vi "tt20panel_DO_apply_settings.vi"(8 "error in (no error)":errorcluster, 10 "tt20_settings":T1, 11 "tt20panel in":refnum<class "tt20panel.lvclass">) -> (0 "error out":errorcluster, 3 "tt20panel out":refnum<class "tt20panel.lvclass">)   [LabVIEW 2015, in "tt20panel.lvclass"]
uses:
  tt20panel.lvclass
  tt20_class/tt20_hardware_info_tdef.ctl
  tt20_acq_mode_tdef.ctl
  tt20_class/tt20.lvclass
  UI/panel_class/panel.lvclass
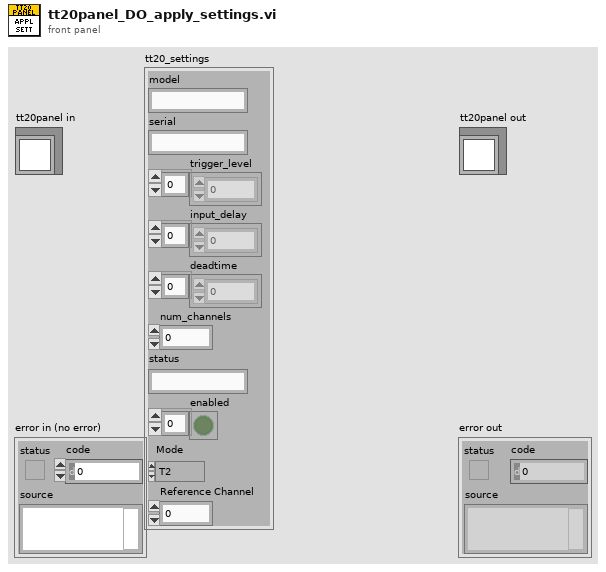
[diagram p1: front panel]
types:
  T1 = typedef "tt20_hardware_info_tdef.ctl" = cluster{"model":string, "serial":string, "trigger_level":dbl[], "input_delay":i64[], "deadtime":i64[], "num_channels":u32, "status":string, "enabled":bool[], "Mode":T2, "Reference Channel":u8}
  T2 = typedef "tt20_acq_mode_tdef.ctl" = enum16{"T2", "T3"}
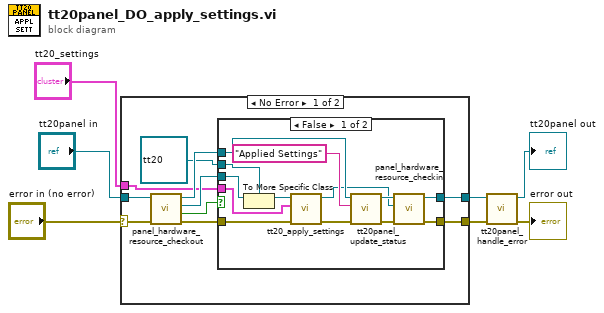
[diagram p0: block diagram]
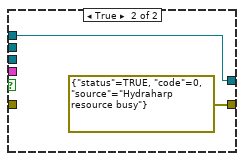
[diagram p2: hidden frame]
diagram:
  n1 = case shown="No Error" "error in (no error)" {
    selector: "error in (no error)" -> [w16 w34]
    tunnel: [w13 w34] -> w5
    tunnel: [w10 w33] -> w2
    tunnel: "tt20panel in" -> [w17 w33]
    tunnel: "tt20_settings" -> [w8 _]
    frame No Error {
      n2 = call "panel_hardware_resource_checkout.vi"("error in (no error)"=w16, "panel in"=w17) -> ("error out"=w14:errorcluster, "timed out?"=w15:bool, "hardware.lvclass"=w11:refnum<class "hardware.lvclass">, "panel out"=w12:refnum<class "tt20panel.lvclass">)  [unwired: 6 in]
      n3 = case shown="False" w15 {
        tunnel: w14 -> [w22 _]
        tunnel: [w28 errorcluster {"status"=TRUE, "code"=0, "source"="Hydraharp resource busy"} ("error out")] -> w13
        tunnel: w12 -> [w26 w31]
        tunnel: w11 -> [w29 _]
        tunnel: refnum<class "tt20.lvclass"> refnum ("tt20.lvclass") -> [w30 _]
        tunnel: [w27 w31] -> w10
        tunnel: w8 -> [w18 _]
        frame False {
          n4 = To More Specific Class(target class=w30, reference=w29) -> (specific class reference=w19:refnum<class "tt20.lvclass">)  [unwired: 1 in, 1 out]
          n5 = call "tt20_apply_settings.vi"("error in (no error)"=w22, "tt20_info"=w18, "tt20 in"=w19) -> ("error out"=w21:errorcluster, "tt20 out"=w20:refnum<class "tt20.lvclass">)  [unwired: 7 in]
          n6 = call "tt20panel_update_status.vi"("error in (no error)"=w21, "status"="Applied Settings", "tt20panel in"=w26) -> ("error out"=w24:errorcluster, "tt20panel out"=w25:refnum<class "tt20panel.lvclass">)  [unwired: 7 in]
          n7 = call "panel_hardware_resource_checkin.vi"("error in (no error)"=w24, "hardware.lvclass"=w20, "panel in"=w25) -> ("error out"=w28:errorcluster, "panel out"=w27:refnum<class "tt20panel.lvclass">)  [unwired: 7 in]
        }
        frame True {
        }
      }
    }
    frame Error {
    }
  }
  n8 = call "tt20panel_handle_error.vi"("error in (no error)"=w5, "tt20panel in"=w2) -> ("error out"=→"error out":errorcluster, "tt20panel out"=→"tt20panel out":refnum<class "tt20panel.lvclass">)  [unwired: 8 in]
